vi "PJ1_work.vi"() -> ()   [LabVIEW 2024]
uses:
  C:/Users/Windows 11/Downloads/Control 9.ctl
  <vilib>/Instr/_visa.llb/VISA Configure Serial Port (Instr).vi
  <vilib>/express/express analysis/Spectral/Block/exnSpectralBlock spectral measurements PSD poly.vi
  <vilib>/express/express analysis/Spectral/Block/exnSpectralBlock spectral measurements PSD DDT.vi
  <vilib>/express/express analysis/Spectral/XNode/ExpressSpectralMeasurementsBlockNode.xnode
panel:
  in  "Upper Cut-Off":dbl=40.0
  out "PSD":dynamicdata(graph)
  out "PSD MAX":dbl
  out "Index ที่มากที่สุด":i32
  out "max value":dbl
  out "B 18+1":dbl
  out "N 18+1":dbl
  in  "Aj 18+1":dbl
  out "B 18+1":dbl
  out "PSD 18+1":dbl
  out "B 18":dbl
  out "N 18":dbl
  in  "Aj 18":dbl
  out "B 18":dbl
  out "PSD 18":dbl
  out "B 18-1":dbl
  out "N 18-1":dbl
  in  "Aj 18-1":dbl
  out "B 18-1":dbl
  out "PSD 18-1":dbl
  out "9 Hz":dbl[](array[numeric])
  out "Max Index 9":i32
  out "PSD max 9":dbl
  out "PSD 9-1":dbl
  out "B 9-1":dbl
  in  "Aj 9-1":dbl
  out "N 9-1":dbl
  out "B 9-1":dbl
  out "PSD 9":dbl
  out "B 9":dbl
  in  "Aj 9":dbl
  out "N 9":dbl
  out "B 9":dbl
  out "PSD 9+1":dbl
  out "B 9+1":dbl
  in  "Aj 9+1":dbl
  out "N 9+1":dbl
  out "B 9+1":dbl
  out "8 Hz":dbl[](array[numeric])
  out "Max Index 8":i32
  out "PSD max 8":dbl
  out "B 16+1":dbl
  out "N 16+1":dbl
  in  "Aj  16+1":dbl
  out "B 16+1":dbl
  out "PSD  16+1":dbl
  out "B 16":dbl
  out "N  16":dbl
  in  "Aj  16":dbl
  out "B 16":dbl
  out "PSD  16":dbl
  out "B 16-1":dbl
  out "N  16-1":dbl
  in  "Aj   16-1":dbl
  out "B   16-1":dbl
  out "PSD 16-1":dbl
  out "B 8+1":dbl
  out "N 8+1":dbl
  in  "Aj  8+1":dbl
  out "B  8+1":dbl
  out "PSD 8+1":dbl
  out "B 8":dbl
  out "N  8":dbl
  in  "Aj  8":dbl
  out "B  8":dbl
  out "PSD 8":dbl
  out "B 8-1":dbl
  out "N  8-1":dbl
  in  "Aj  8-1":dbl
  out "B  8-1":dbl
  out "PSD 8-1":dbl
  out "PSD 14+1":dbl
  out "B 14+1":dbl
  in  "Aj 14+1":dbl
  out "N 14+1":dbl
  out "B 14+1":dbl
  out "PSD 14":dbl
  out "B 14":dbl
  in  "Aj 14":dbl
  out "N 14":dbl
  out "B 14":dbl
  out "PSD 14-1":dbl
  out "B 14-1":dbl
  in  "Aj 14-1":dbl
  out "N 14-1":dbl
  out "B 14-1":dbl
  out "PSD7+1":dbl
  out "B7+1":dbl
  in  "Aj7+1":dbl
  out "N7+1":dbl
  out "B7+1":dbl
  out "PSD 7":dbl
  out "B 7":dbl
  in  "Aj 7":dbl
  out "N7":dbl
  out "B7":dbl
  out "7 Hz":dbl[](array[numeric])
  out "Max Index 7":i32
  out "PSD max 7":dbl
  out "PSD 7-1":dbl
  out "B 7-1":dbl
  in  "Aj 7-1":dbl
  out "N7-1":dbl
  out "B7-1":dbl
  out "B12-1":dbl
  out "N12-1":dbl
  in  "Aj 12-1":dbl
  out "B 12-1":dbl
  out "PSD 12-1":dbl
  out "B12":dbl
  out "N12":dbl
  in  "Aj 12":dbl
  out "B12":dbl
  out "PSD 12":dbl
  out "B12+1":dbl
  out "N12+1":dbl
  in  "Aj 12+1":dbl
  out "B 12+1":dbl
  out "PSD 12+1":dbl
  out "B6+1":dbl
  out "N6+1":dbl
  in  "Aj 6+1":dbl
  out "B 6+1":dbl
  out "PSD 6+1":dbl
  out "B6":dbl
  out "N6":dbl
  in  "Aj 6":dbl
  out "B6":dbl
  out "PSD 6":dbl
  out "PSD 6-1":dbl
  out "6 Hz":dbl[](array[numeric])
  out "Max Index 6":i32
  out "PSD max 6":dbl
  out "B 6-1":dbl
  in  "Aj 6-1":dbl
  out "N6-1":dbl
  out "B6-1":dbl
  in  "Baseline":bool
  out "appended array":dbl[][](array[numeric])
  out "Filtered Signal":dynamicdata(graph)
  in  "Lower Cut-Off":dbl=1.0
  out "data":dynamicdata(graph) caption="Raw Data"
  in  "number of samples":i32=1000
  in  "rate":dbl=200.0 min=200.0 max=200.0
  out "?":bool
  out "?":bool
  out "?":bool
  out "?":bool
  out "?":bool
  out "?":bool
  out "?":bool
  out "?":bool
  out "?":bool
  out "?":bool
  out "?":bool=TRUE
  out "?":bool=TRUE
  out "?":bool=TRUE
  out "?":bool=TRUE
  out "?":bool=TRUE
  out "?":bool=TRUE
  out "?":bool=TRUE
  out "?":bool=TRUE
  out "?":bool=TRUE
  out "?":bool=TRUE
  out "?":bool
  out "?":bool
  out "?":bool
  out "?":bool
  out "?":bool
  out "?":bool
  out "?":bool
  out "?":bool
  out "?":bool
  out "?":bool
  out "?":bool=TRUE
  out "?":bool=TRUE
  out "?":bool=TRUE
  out "?":bool=TRUE
  out "?":bool=TRUE
  out "?":bool=TRUE
  out "?":bool=TRUE
  out "?":bool=TRUE
  out "?":bool=TRUE
  out "?":bool=TRUE
  out "?":bool
  out "?":bool
  out "?":bool
  out "?":bool
  out "?":bool
  out "?":bool
  out "?":bool
  out "?":bool
  out "?":bool
  out "?":bool
  out "?":bool=TRUE
  out "?":bool=TRUE
  out "?":bool=TRUE
  out "?":bool=TRUE
  out "?":bool=TRUE
  out "?":bool=TRUE
  out "?":bool=TRUE
  out "?":bool=TRUE
  out "?":bool=TRUE
  out "?":bool=TRUE
  out "?":bool
  out "?":bool
  out "?":bool
  out "?":bool
  out "?":bool
  out "?":bool
  out "?":bool
  out "?":bool
  out "?":bool
  out "?":bool
  out "?":bool=TRUE
  out "?":bool=TRUE
  out "?":bool=TRUE
  out "?":bool=TRUE
  out "?":bool=TRUE
  out "?":bool=TRUE
  out "?":bool=TRUE
  out "?":bool=TRUE
  out "?":bool=TRUE
  out "?":bool=TRUE
  out "9 HZ":bool
  out "8 HZ":bool
  out "6 HZ":bool
  out "7 HZ":bool
  in  "Tab Control":enum32{"TAB 1", "TAB 2", "TAB 3", "TAB 4"}(tab)
  out "555":bool
  in  "MENU 4":bool
  in  "MENU 3":bool
  in  "MENU 2":bool
  in  "MENU":bool
  in  "start":bool
  in  "Text3":bool
  in  "Text2":bool
  in  "Backpage 2":T1
  out "String":string
  in  "Text1":bool
  in  "send":bool
  in  "Back":bool
  in  "1 3":bool
  in  "1 2":bool
  in  "1":bool
  out "String 2":string
  in  "SOS CALLING":bool
  in  "Blank Button 14":bool
  in  "LED":bool
  in  "Blank Button 12":bool
  in  "Back 4":bool
  in  "VISA resource name":refnum<visa-resource-name>
  # "Tel."
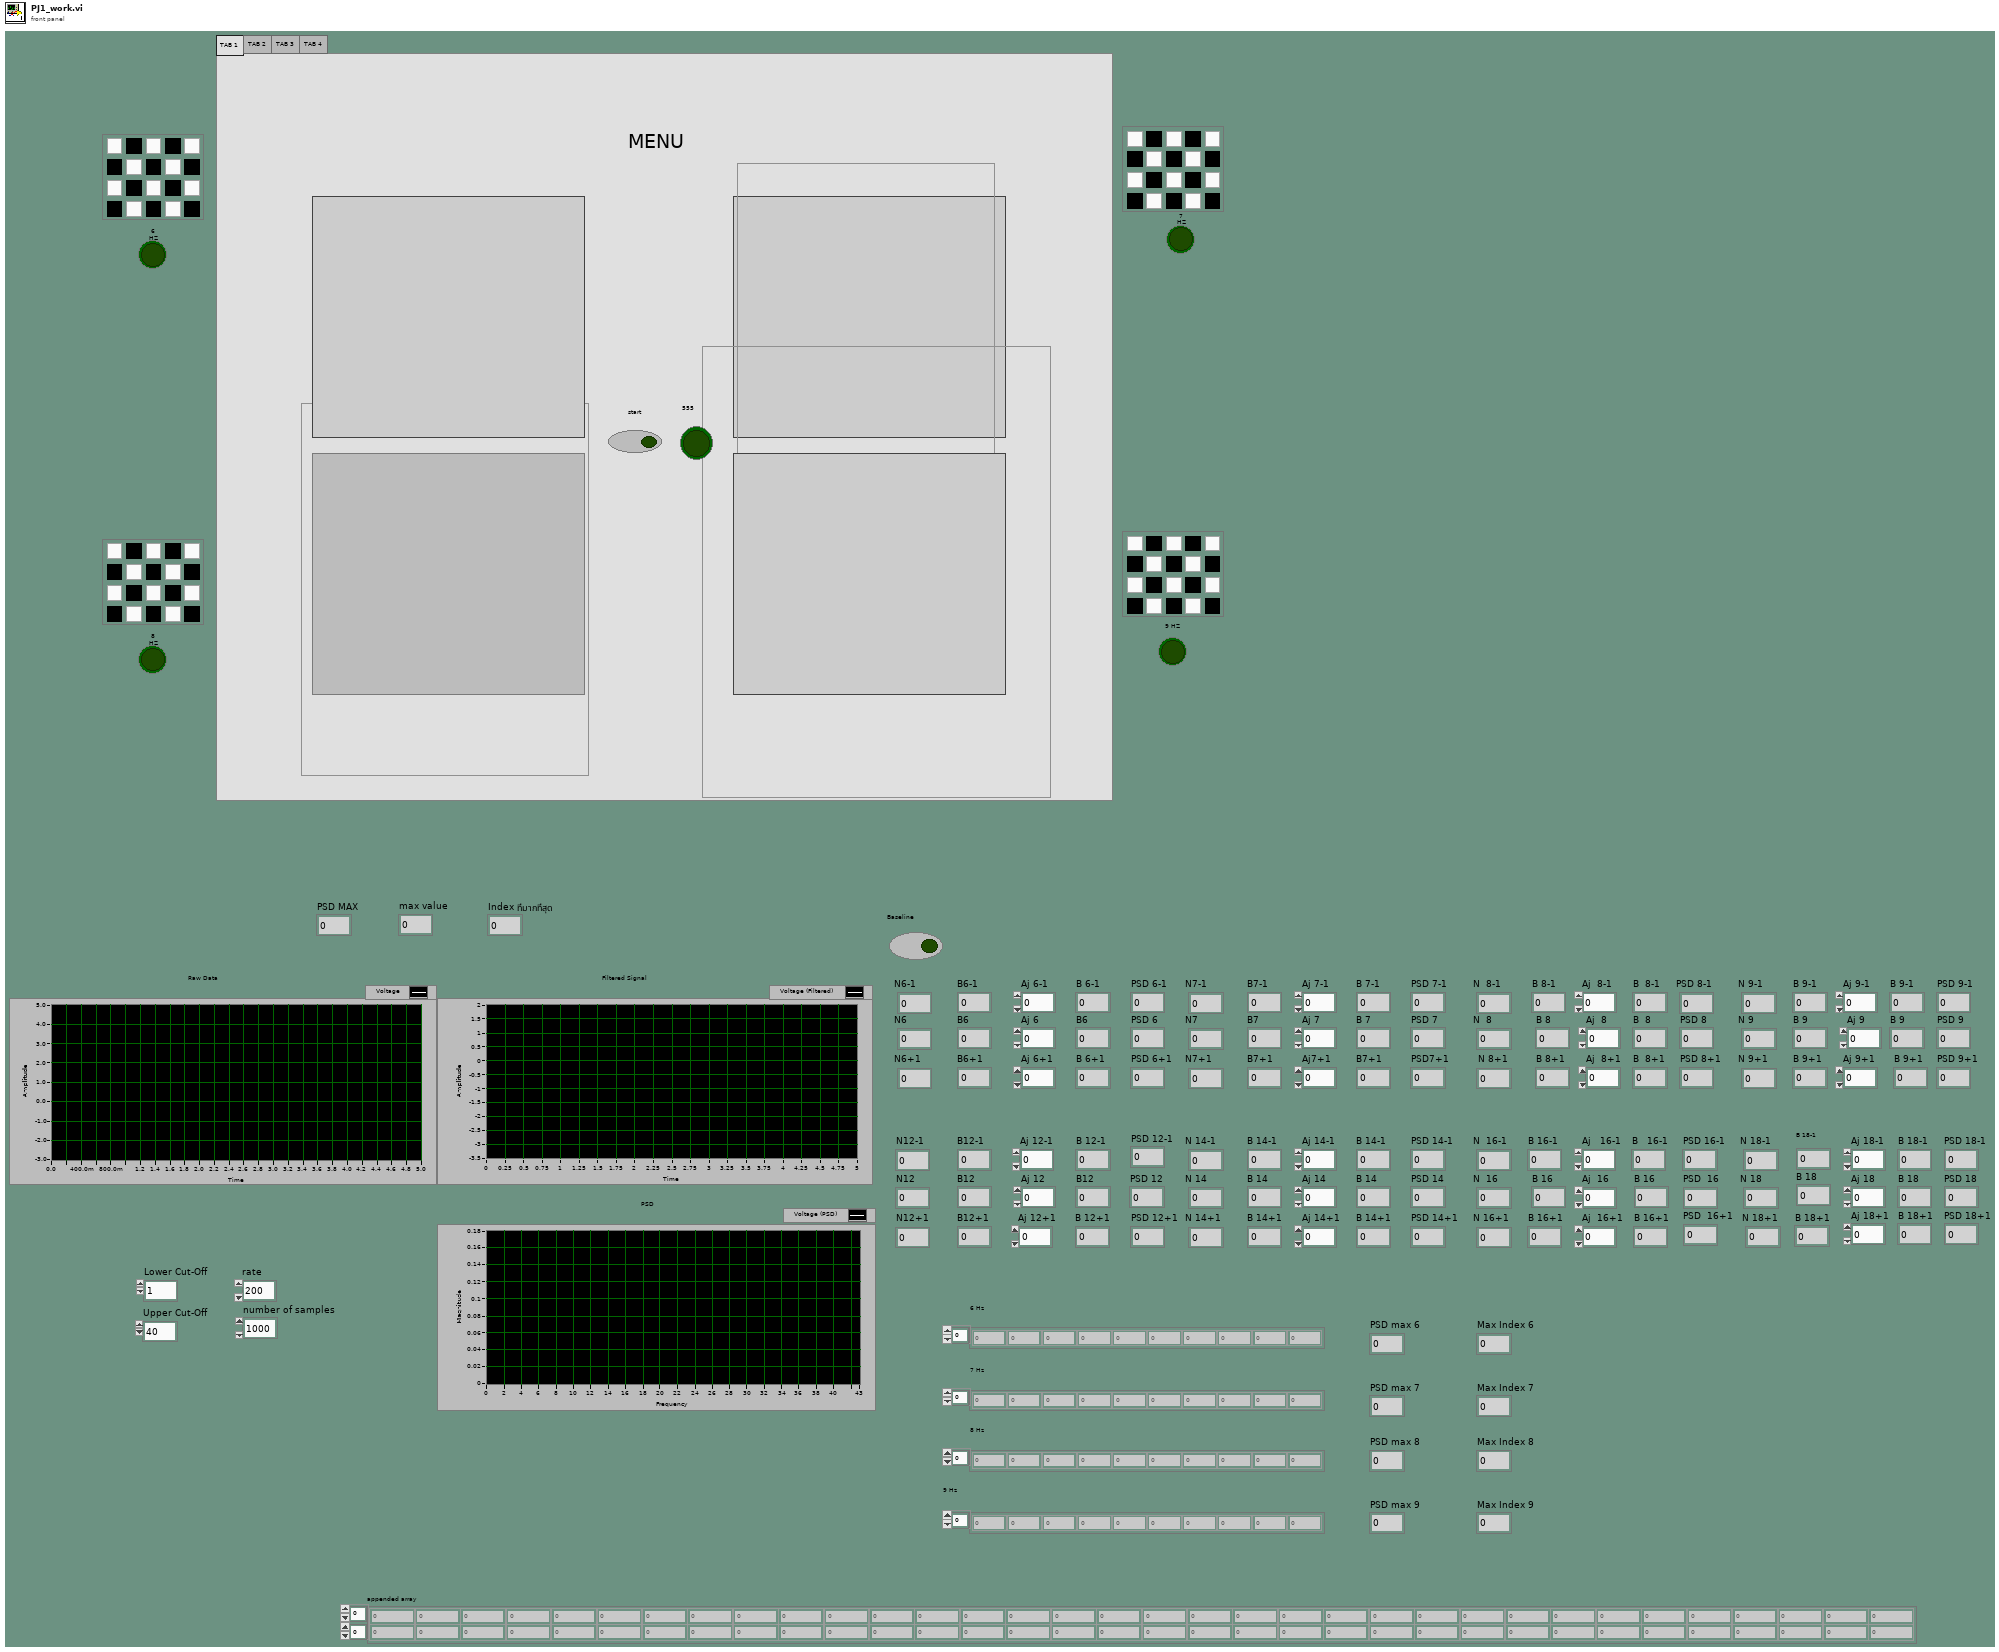
[diagram p1: front panel]
types:
  T1 = typedef "Control 9.ctl" = bool
  T2 = cluster{"averaging mode":u16, "weighting mode":u16, "number of averages":u32}
  T3 = cluster{"dB On (F)":bool, "unwrap phase (F)":bool, "convert to degree (F)":bool}
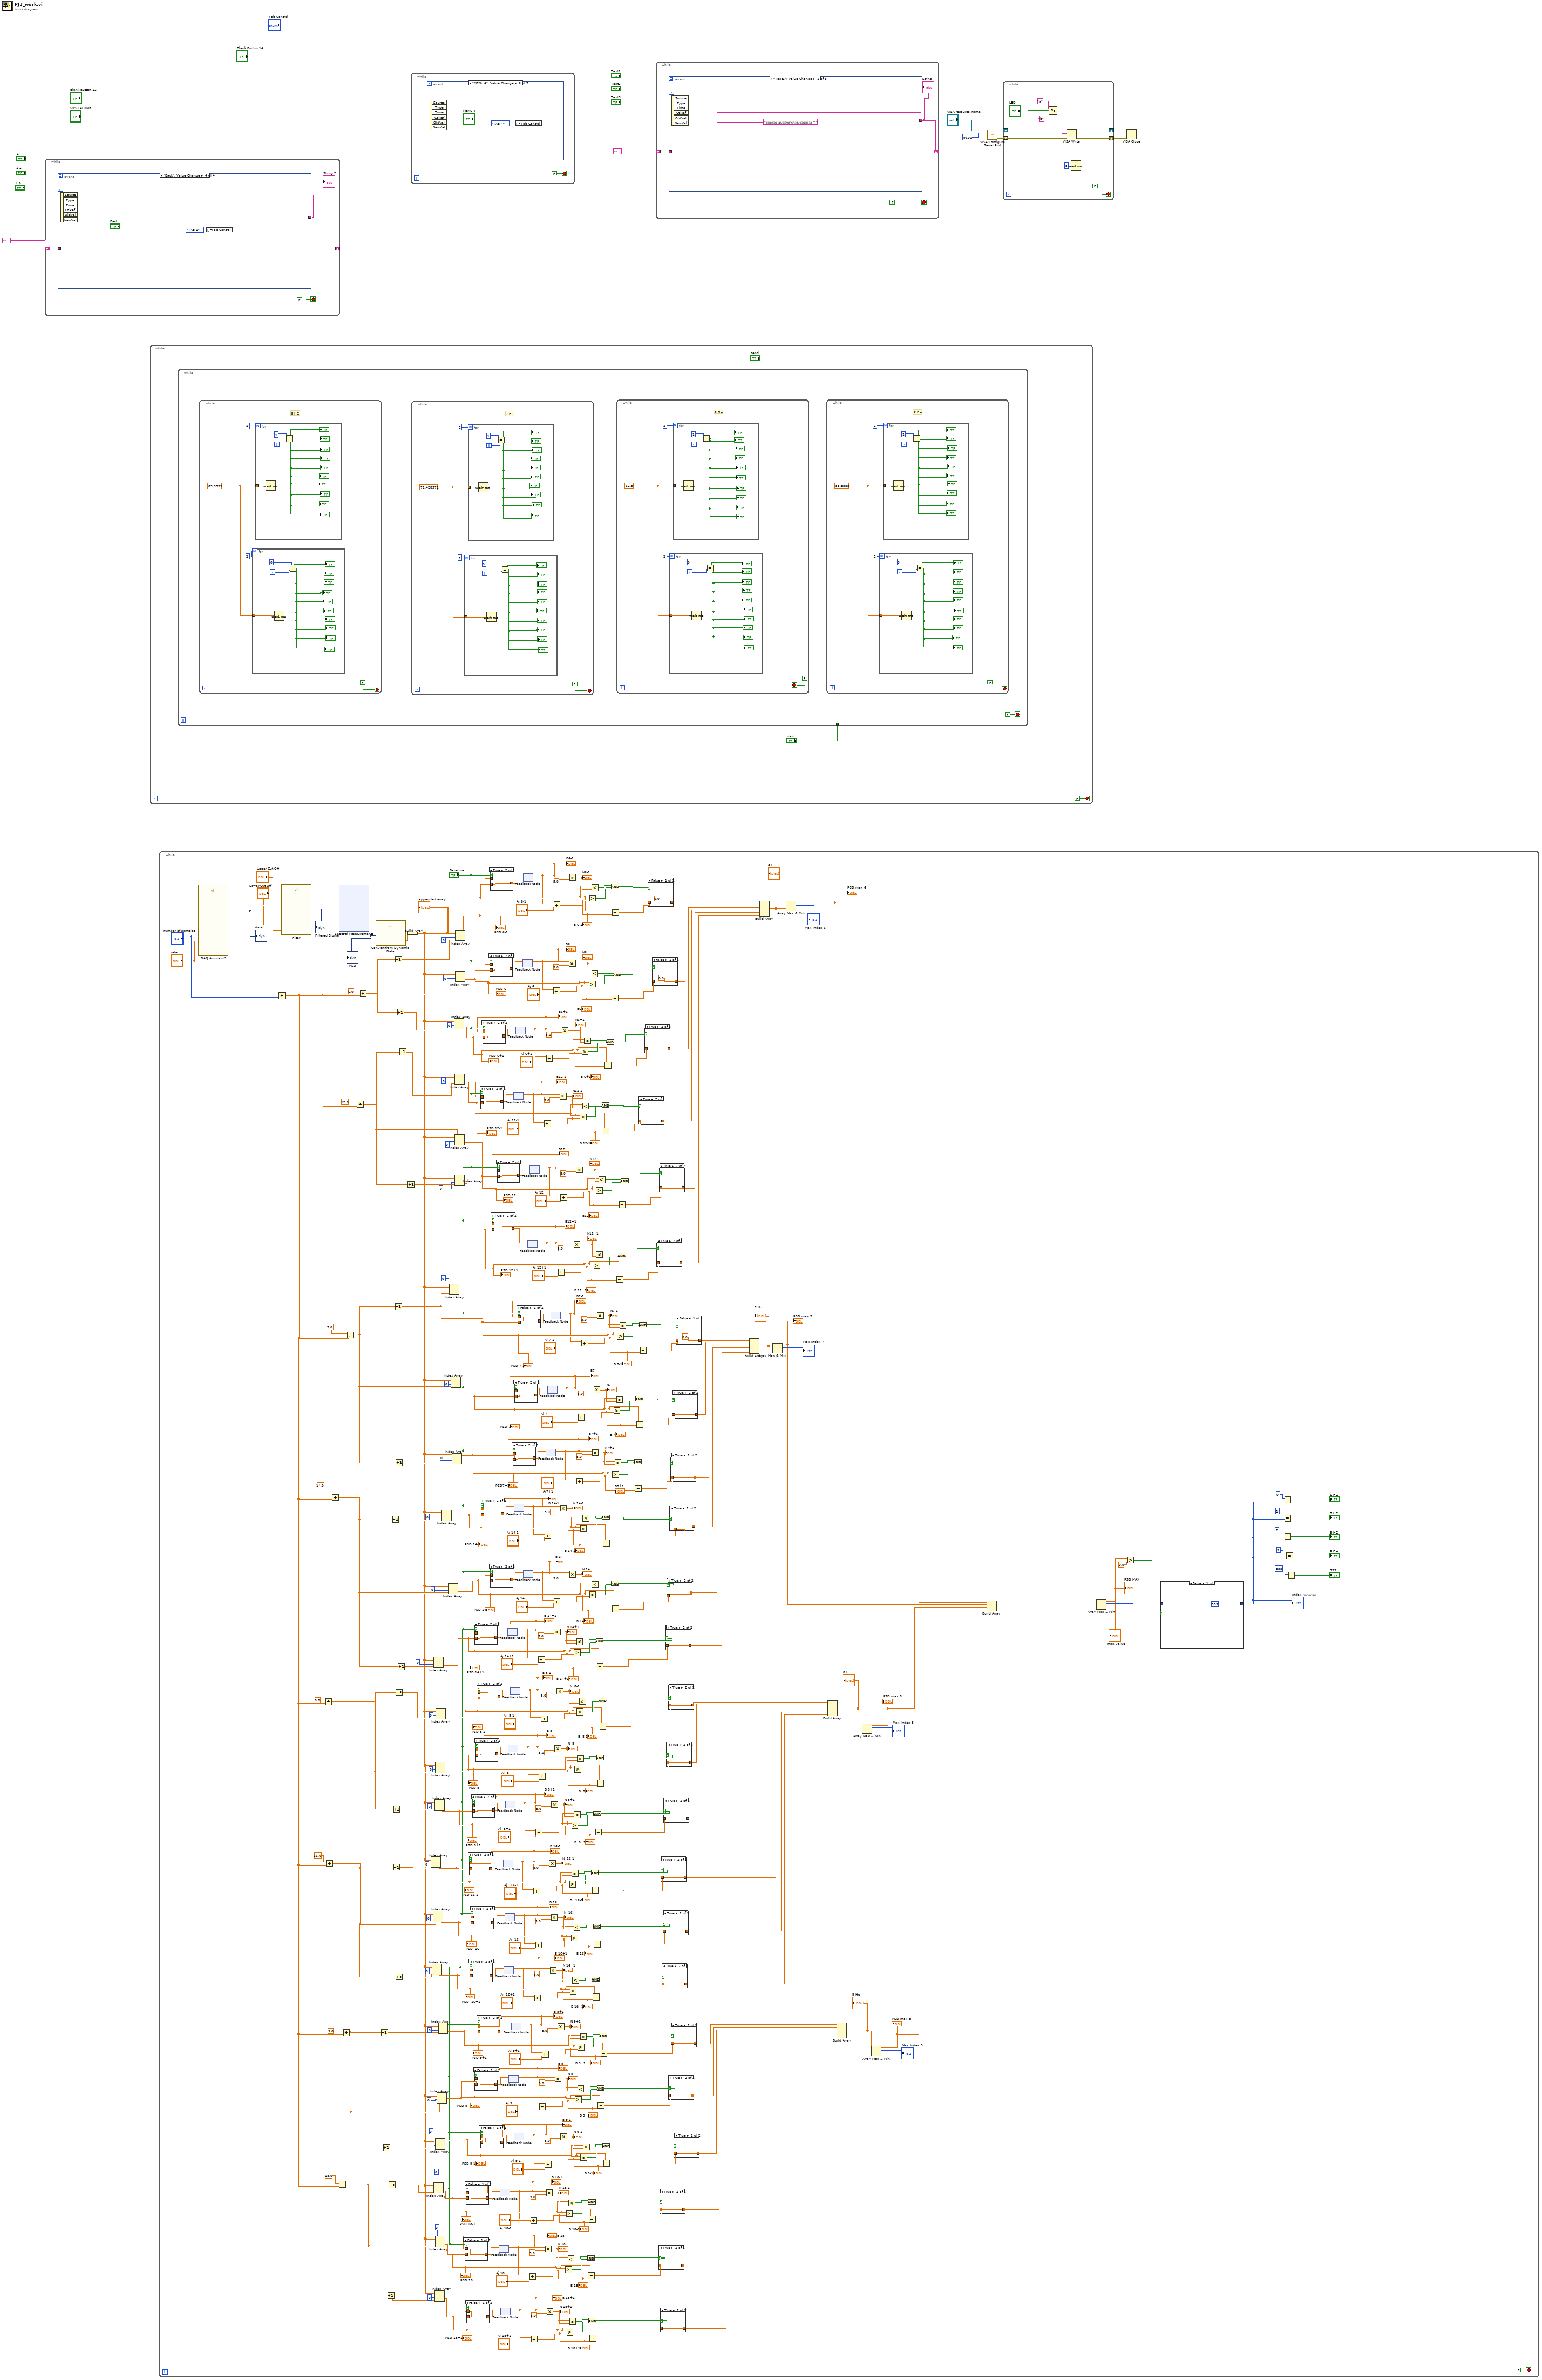
[diagram p0: block diagram]
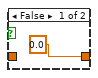
[diagram p3: hidden frame]
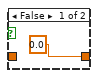
[diagram p5: hidden frame]
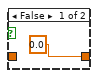
[diagram p7: hidden frame]
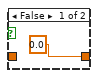
[diagram p9: hidden frame]
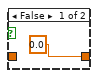
[diagram p11: hidden frame]
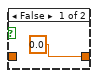
[diagram p13: hidden frame]
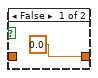
[diagram p15: hidden frame]
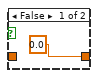
[diagram p17: hidden frame]
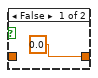
[diagram p19: hidden frame]
diagram:
  n1 = while {
    shift-right: [w9] -> _
    shift-left: "" -> [w11]
    stop <- FALSE stop-if-true
    n2 = event shown="[3] \"Back\": Value Change" {
      selector: _ -> [_ _ _ _]
      dyn-events: _ -> [_ _ _ _]
      timeout: _ -> [_ _ _ _]
      tunnel: w11 -> [_ _ _ _]
      tunnel: ["0622436287" "1669" " 0937529340" _] -> w9
      event "1 2": Value Change {
        n3 = event-data() -> ()  [unwired: 1 in, 6 out]
      }
      event "1": Value Change {
        n4 = event-data() -> ()  [unwired: 1 in, 6 out]
      }
      event "1 3": Value Change {
        n5 = event-data() -> ()  [unwired: 1 in, 6 out]
      }
      event "Back": Value Change {
        n6 = event-data() -> ()  [unwired: 1 in, 6 out]
        n7 = local write "Tab Control"(enum32{"TAB 1", "TAB 2", "TAB 3", "TAB 4"}."TAB 1" ("Tab Control")) -> ()
      }
    }
    "String 2" <- w9
  }
  n8 = while {
    stop <- FALSE stop-if-true
    n9 = while {
      tunnel: "start" -> [_]
      stop <- FALSE stop-if-true
      n10 = while {
        stop <- FALSE stop-if-true
        w56 = 83.3333
        # "6 HZ"
        n11 = for {
          N: 2 -> [_]
          tunnel: w56 -> [w60]
          i -> [w62]
          n12 = Wait (ms)(milliseconds to wait=w60) -> ()  [unwired: 1 out]
          n13 = Equal?(x=0, y=w62) -> (x = y?=→"?" →"?" →"?" →"?" →"?" →"?" →"?" →"?" →"?" →"?":bool)
        }
        n14 = for {
          N: 2 -> [_]
          tunnel: w56 -> [w64]
          i -> [w65]
          n15 = Wait (ms)(milliseconds to wait=w64) -> ()  [unwired: 1 out]
          n16 = Equal?(x=1, y=w65) -> (x = y?=→"?" →"?" →"?" →"?" →"?" →"?" →"?" →"?" →"?" →"?":bool)
        }
      }
      n17 = while {
        stop <- FALSE stop-if-true
        w44 = 71.428571
        # "7 HZ"
        n18 = for {
          N: 2 -> [_]
          tunnel: w44 -> [w48]
          i -> [w50]
          n19 = Wait (ms)(milliseconds to wait=w48) -> ()  [unwired: 1 out]
          n20 = Equal?(x=0, y=w50) -> (x = y?=→"?" →"?" →"?" →"?" →"?" →"?" →"?" →"?" →"?" →"?":bool)
        }
        n21 = for {
          N: 2 -> [_]
          tunnel: w44 -> [w52]
          i -> [w53]
          n22 = Wait (ms)(milliseconds to wait=w52) -> ()  [unwired: 1 out]
          n23 = Equal?(x=1, y=w53) -> (x = y?=→"?" →"?" →"?" →"?" →"?" →"?" →"?" →"?" →"?" →"?":bool)
        }
      }
      n24 = while {
        stop <- FALSE stop-if-true
        w32 = 62.5
        # "8 HZ"
        n25 = for {
          N: 2 -> [_]
          tunnel: w32 -> [w36]
          i -> [w38]
          n26 = Wait (ms)(milliseconds to wait=w36) -> ()  [unwired: 1 out]
          n27 = Equal?(x=0, y=w38) -> (x = y?=→"?" →"?" →"?" →"?" →"?" →"?" →"?" →"?" →"?" →"?":bool)
        }
        n28 = for {
          N: 2 -> [_]
          tunnel: w32 -> [w40]
          i -> [w41]
          n29 = Wait (ms)(milliseconds to wait=w40) -> ()  [unwired: 1 out]
          n30 = Equal?(x=1, y=w41) -> (x = y?=→"?" →"?" →"?" →"?" →"?" →"?" →"?" →"?" →"?" →"?":bool)
        }
      }
      n31 = while {
        stop <- FALSE stop-if-true
        w20 = 55.5555
        # "9 HZ"
        n32 = for {
          N: 2 -> [_]
          tunnel: w20 -> [w24]
          i -> [w26]
          n33 = Wait (ms)(milliseconds to wait=w24) -> ()  [unwired: 1 out]
          n34 = Equal?(x=0, y=w26) -> (x = y?=→"?" →"?" →"?" →"?" →"?" →"?" →"?" →"?" →"?" →"?":bool)
        }
        n35 = for {
          N: 2 -> [_]
          tunnel: w20 -> [w28]
          i -> [w29]
          n36 = Wait (ms)(milliseconds to wait=w28) -> ()  [unwired: 1 out]
          n37 = Equal?(x=1, y=w29) -> (x = y?=→"?" →"?" →"?" →"?" →"?" →"?" →"?" →"?" →"?" →"?":bool)
        }
      }
    }
  }
  n38 = while {
    stop <- FALSE stop-if-true
    n39 = call "DAQ Assistant2"("rate"="rate", "number of samples"="number of samples") -> ("data"=w449:dynamicdata)  [unwired: 15 in, 2 out]
    "data" <- w449
    n40 = Divide(x="rate", y="number of samples") -> (x/y=w156:dbl)
    n41 = call "Filter"("Lower Cut-Off"="Lower Cut-Off", "Upper Cut-Off"="Upper Cut-Off", "Signal"=w449) -> ("Filtered Signal"=w447:dynamicdata)  [unwired: 7 in, 1 out]
    "Filtered Signal" <- w447
    n42 = Divide(x=8.0, y=w156) -> (x/y=w256:dbl)
    n43 = Divide(x=16.0, y=w156) -> (x/y=w208:dbl)
    n44 = Divide(x=14.0, y=w156) -> (x/y=w281:dbl)
    n45 = Divide(x=18.0, y=w156) -> (x/y=w131:dbl)
    n46 = xnode "Spectral Measurements"("Signals"=w447) -> ("PSD"=w93:dynamicdata)  [unwired: 1 in, 1 out]
    "PSD" <- w93
    n47 = Divide(x=9.0, y=w156) -> (x/y=w174:dbl)
    n48 = Divide(x=7.0, y=w156) -> (x/y=w298:dbl)
    n49 = Divide(x=12.0, y=w156) -> (x/y=w367:dbl)
    n50 = Divide(x=6.0, y=w156) -> (x/y=w416:dbl)
    n51 = call "Convert from Dynamic Data"("Dynamic Data Type"=w93) -> ("Array"=w446:dbl[])  [unwired: 3 in]
    n52 = Decrement(x=w174) -> (x-1=w205:dbl)
    n53 = Increment(x=w174) -> (x+1=w173:dbl)
    n54 = Increment(x=w131) -> (x+1=w120:dbl)
    n55 = Decrement(x=w131) -> (x-1=w145:dbl)
    n56 = Decrement(x=w281) -> (x-1=w310:dbl)
    n57 = Increment(x=w256) -> (x+1=w246:dbl)
    n58 = Decrement(x=w208) -> (x-1=w231:dbl)
    n59 = Decrement(x=w416) -> (x-1=w429:dbl)
    n60 = Decrement(x=w298) -> (x-1=w339:dbl)
    "PSD 7-1" <- w339
    n61 = Increment(x=w298) -> (x+1=w324:dbl)
    n62 = Decrement(x=w256) -> (x-1=w269:dbl)
    n63 = Increment(x=w208) -> (x+1=w207:dbl)
    n64 = Increment(x=w416) -> (x+1=w405:dbl)
    n65 = Increment(x=w281) -> (x+1=w287:dbl)
    n66 = Decrement(x=w367) -> (x-1=w372:dbl)
    n67 = Increment(x=w367) -> (x+1=w366:dbl)
    n68 = Build Array(w446) -> (w121:dbl[][])
    "appended array" <- w121
    n69 = Index Array(array=w121, index (row)=0, index (col)=w231) -> (element=w242:dbl)
    "PSD 16-1" <- w242
    n70 = Index Array(array=w121, index (row)=0 ("disabled index (row)"), index (col)=w207) -> (element=w219:dbl)
    "PSD  16+1" <- w219
    n71 = Index Array(array=w121, index (row)=0 ("disabled index (row)"), index (col)=w208) -> (element=w221:dbl)
    "PSD  16" <- w221
    n72 = Index Array(array=w121, index (row)=0, index (col)=w287) -> (element=w288:dbl)
    "PSD 14+1" <- w288
    n73 = Index Array(array=w121, index (row)=0 ("disabled index (row)"), index (col)=w145) -> (element=w143:dbl)
    "PSD 18-1" <- w143
    n74 = Index Array(array=w121, index (row)=0, index (col)=w246) -> (element=w244:dbl)
    "PSD 8+1" <- w244
    n75 = Index Array(array=w121, index (row)=0 ("disabled index (row)"), index (col)=w120) -> (element=w117:dbl)
    "PSD 18+1" <- w117
    n76 = Index Array(array=w121, index (row)=0, index (col)=w173) -> (element=w162:dbl)
    "PSD 9-1" <- w162
    n77 = Index Array(array=w121, index (row)=0, index (col)=w256) -> (element=w267:dbl)
    "PSD 8" <- w267
    n78 = Index Array(array=w121, index (row)=0 ("disabled index (row)"), index (col)=w131) -> (element=w132:dbl)
    "PSD 18" <- w132
    n79 = Index Array(array=w121, index (row)=0, index (col)=w269) -> (element=w268:dbl)
    "PSD 8-1" <- w268
    n80 = Index Array(array=w121, index (row)=0, index (col)=w174) -> (element=w175:dbl)
    "PSD 9" <- w175
    n81 = Index Array(array=w121, index (row)=0, index (col)=w205) -> (element=w186:dbl)
    "PSD 9+1" <- w186
    n82 = Index Array(array=w121, index (row)=0, index (col)=w310) -> (element=w312:dbl)
    "PSD 14-1" <- w312
    n83 = Index Array(array=w121, index (row)=0, index (col)=w281) -> (element=w299:dbl)
    "PSD 14" <- w299
    n84 = Index Array(array=w121, index (row)=0, index (col)=w339) -> ()  [unwired: 1 out]
    n85 = Index Array(array=w121, index (row)=0 ("disabled index (row)"), index (col)=w298) -> (element=w336:dbl)
    "PSD 7" <- w336
    n86 = Index Array(array=w121, index (row)=0, index (col)=w324) -> (element=w325:dbl)
    "PSD7+1" <- w325
    n87 = Index Array(array=w121, index (row)=0 ("disabled index (row)"), index (col)=w405) -> (element=w403:dbl)
    "PSD 6+1" <- w403
    n88 = Index Array(array=w121, index (row)=0, index (col)=w372) -> (element=w371:dbl)
    "PSD 12-1" <- w371
    n89 = Index Array(array=w121, index (row)=0 ("disabled index (row)"), index (col)=w367) -> (element=w368:dbl)
    "PSD 12" <- w368
    n90 = Index Array(array=w121, index (row)=0 ("disabled index (row)"), index (col)=w366) -> (element=w364:dbl)
    "PSD 12+1" <- w364
    n91 = Index Array(array=w121, index (row)=0, index (col)=w416) -> (element=w417:dbl)
    "PSD 6" <- w417
    n92 = Index Array(array=w121, index (row)=0, index (col)=w429) -> (element=w436:dbl)
    "PSD 6-1" <- w436
    n93 = feedback #1() -> (w69:dbl)  [unwired: 1 in]
    "B 18" <- w69
    n94 = case shown="False" "Baseline" {
      tunnel: w132 -> [_ w459]
      tunnel: [w458 w459] -> w134
      tunnel: w69 -> [w458 _]
      frame False {
      }
      frame True {
      }
    }
    n95 = feedback-in #1(w134) -> ()
    n96 = feedback #2() -> (w70:dbl)  [unwired: 1 in]
    "B 18-1" <- w70
    n97 = case shown="False" "Baseline" {
      tunnel: w143 -> [_ w463]
      tunnel: [w462 w463] -> w154
      tunnel: w70 -> [w462 _]
      frame False {
      }
      frame True {
      }
    }
    n98 = feedback-in #2(w154) -> ()
    n99 = feedback #3() -> (w68:dbl)  [unwired: 1 in]
    "B 18+1" <- w68
    n100 = case shown="False" "Baseline" {
      tunnel: w117 -> [_ w455]
      tunnel: [w454 w455] -> w130
      tunnel: w68 -> [w454 _]
      frame False {
      }
      frame True {
      }
    }
    n101 = feedback-in #3(w130) -> ()
    n102 = feedback #4() -> (w76:dbl)  [unwired: 1 in]
    "B 16-1" <- w76
    n103 = case shown="True" "Baseline" {
      tunnel: w242 -> [_ w487]
      tunnel: [w486 w487] -> w232
      tunnel: w76 -> [w486 _]
      frame False {
      }
      frame True {
      }
    }
    n104 = feedback-in #4(w232) -> ()
    n105 = feedback #5() -> (w74:dbl)  [unwired: 1 in]
    "B 16+1" <- w74
    n106 = case shown="True" "Baseline" {
      tunnel: w219 -> [_ w479]
      tunnel: [w478 w479] -> w210
      tunnel: w74 -> [w478 _]
      frame False {
      }
      frame True {
      }
    }
    n107 = feedback-in #5(w210) -> ()
    n108 = feedback #6() -> (w75:dbl)  [unwired: 1 in]
    "B 16" <- w75
    n109 = case shown="True" "Baseline" {
      tunnel: w221 -> [_ w483]
      tunnel: [w482 w483] -> w230
      tunnel: w75 -> [w482 _]
      frame False {
      }
      frame True {
      }
    }
    n110 = feedback-in #6(w230) -> ()
    n111 = feedback #7() -> (w77:dbl)  [unwired: 1 in]
    "B 8+1" <- w77
    n112 = case shown="True" "Baseline" {
      tunnel: w244 -> [_ w491]
      tunnel: [w490 w491] -> w255
      tunnel: w77 -> [w490 _]
      frame False {
      }
      frame True {
      }
    }
    n113 = feedback-in #7(w255) -> ()
    n114 = feedback #8() -> (w80:dbl)  [unwired: 1 in]
    "B 14+1" <- w80
    n115 = case shown="True" "Baseline" {
      tunnel: w288 -> [_ w503]
      tunnel: [w502 w503] -> w289
      tunnel: w80 -> [w502 _]
      frame False {
      }
      frame True {
      }
    }
    n116 = feedback-in #8(w289) -> ()
    n117 = feedback #9() -> (w78:dbl)  [unwired: 1 in]
    "B 8" <- w78
    n118 = case shown="True" "Baseline" {
      tunnel: w267 -> [_ w495]
      tunnel: [w494 w495] -> w258
      tunnel: w78 -> [w494 _]
      frame False {
      }
      frame True {
      }
    }
    n119 = feedback-in #9(w258) -> ()
    n120 = feedback #10() -> (w72:dbl)  [unwired: 1 in]
    "B 9" <- w72
    n121 = case shown="False" "Baseline" {
      tunnel: w175 -> [_ w471]
      tunnel: [w470 w471] -> w176
      tunnel: w72 -> [w470 _]
      frame False {
      }
      frame True {
      }
    }
    n122 = feedback-in #10(w176) -> ()
    n123 = feedback #11() -> (w79:dbl)  [unwired: 1 in]
    "B 8-1" <- w79
    n124 = case shown="True" "Baseline" {
      tunnel: w268 -> [_ w499]
      tunnel: [w498 w499] -> w279
      tunnel: w79 -> [w498 _]
      frame False {
      }
      frame True {
      }
    }
    n125 = feedback-in #11(w279) -> ()
    n126 = feedback #12() -> (w73:dbl)  [unwired: 1 in]
    "B 9+1" <- w73
    n127 = case shown="True" "Baseline" {
      tunnel: w186 -> [_ w475]
      tunnel: [w474 w475] -> w187
      tunnel: w73 -> [w474 _]
      frame False {
      }
      frame True {
      }
    }
    n128 = feedback-in #12(w187) -> ()
    n129 = feedback #13() -> (w88:dbl)  [unwired: 1 in]
    "B12-1" <- w88
    n130 = case shown="True" "Baseline" {
      tunnel: w371 -> [_ w535]
      tunnel: [w534 w535] -> w383
      tunnel: w88 -> [w534 _]
      frame False {
      }
      frame True {
      }
    }
    n131 = feedback-in #13(w383) -> ()
    n132 = feedback #14() -> (w82:dbl)  [unwired: 1 in]
    "B 14-1" <- w82
    n133 = case shown="True" "Baseline" {
      tunnel: w312 -> [_ w511]
      tunnel: [w510 w511] -> w313
      tunnel: w82 -> [w510 _]
      frame False {
      }
      frame True {
      }
    }
    n134 = feedback-in #14(w313) -> ()
    n135 = feedback #15() -> (w71:dbl)  [unwired: 1 in]
    "B 9-1" <- w71
    n136 = case shown="False" "Baseline" {
      tunnel: w162 -> [_ w467]
      tunnel: [w466 w467] -> w163
      tunnel: w71 -> [w466 _]
      frame False {
      }
      frame True {
      }
    }
    n137 = feedback-in #15(w163) -> ()
    n138 = feedback #16() -> (w89:dbl)  [unwired: 1 in]
    "B6+1" <- w89
    n139 = case shown="True" "Baseline" {
      tunnel: w403 -> [_ w539]
      tunnel: [w538 w539] -> w406
      tunnel: w89 -> [w538 _]
      frame False {
      }
      frame True {
      }
    }
    n140 = feedback-in #16(w406) -> ()
    n141 = feedback #17() -> (w90:dbl)  [unwired: 1 in]
    "B6" <- w90
    n142 = case shown="True" "Baseline" {
      tunnel: w417 -> [_ w543]
      tunnel: [w542 w543] -> w427
      tunnel: w90 -> [w542 _]
      frame False {
      }
      frame True {
      }
    }
    n143 = feedback-in #17(w427) -> ()
    n144 = feedback #18() -> (w91:dbl)  [unwired: 1 in]
    "B6-1" <- w91
    n145 = case shown="True" "Baseline" {
      tunnel: w436 -> [_ w547]
      tunnel: [w546 w547] -> w428
      tunnel: w91 -> [w546 _]
      frame False {
      }
      frame True {
      }
    }
    n146 = feedback-in #18(w428) -> ()
    n147 = feedback #19() -> (w81:dbl)  [unwired: 1 in]
    "B 14" <- w81
    n148 = case shown="True" "Baseline" {
      tunnel: w299 -> [_ w507]
      tunnel: [w506 w507] -> w301
      tunnel: w81 -> [w506 _]
      frame False {
      }
      frame True {
      }
    }
    n149 = feedback-in #19(w301) -> ()
    n150 = feedback #20() -> (w86:dbl)  [unwired: 1 in]
    "B12+1" <- w86
    n151 = case shown="True" "Baseline" {
      tunnel: w364 -> [_ w527]
      tunnel: [w526 w527] -> w401
      tunnel: w86 -> [w526 _]
      frame False {
      }
      frame True {
      }
    }
    n152 = feedback-in #20(w401) -> ()
    n153 = Add(x=w69, y="Aj 18") -> (x+y=w138:dbl)
    "B 18" <- w138
    n154 = Add(x=w70, y="Aj 18-1") -> (x+y=w150:dbl)
    "B 18-1" <- w150
    n155 = Add(x=w68, y="Aj 18+1") -> (x+y=w126:dbl)
    "B 18+1" <- w126
    n156 = feedback #21() -> (w87:dbl)  [unwired: 1 in]
    "B12" <- w87
    n157 = case shown="True" "Baseline" {
      tunnel: w368 -> [_ w531]
      tunnel: [w530 w531] -> w384
      tunnel: w87 -> [w530 _]
      frame False {
      }
      frame True {
      }
    }
    n158 = feedback-in #21(w384) -> ()
    n159 = Add(x=w76, y="Aj   16-1") -> (x+y=w236:dbl)
    "B   16-1" <- w236
    n160 = Add(x=w74, y="Aj  16+1") -> (x+y=w214:dbl)
    "B 16+1" <- w214
    n161 = Add(x=w75, y="Aj  16") -> (x+y=w226:dbl)
    "B 16" <- w226
    n162 = Add(x=w77, y="Aj  8+1") -> (x+y=w251:dbl)
    "B  8+1" <- w251
    n163 = Add(x=w80, y="Aj 14+1") -> (x+y=w293:dbl)
    "B 14+1" <- w293
    n164 = Add(x=w78, y="Aj  8") -> (x+y=w262:dbl)
    "B  8" <- w262
    n165 = Add(x=w72, y="Aj 9") -> (x+y=w180:dbl)
    "B 9" <- w180
    n166 = Add(x=w79, y="Aj  8-1") -> (x+y=w275:dbl)
    "B  8-1" <- w275
    n167 = Add(x=w73, y="Aj 9+1") -> (x+y=w191:dbl)
    "B 9+1" <- w191
    n168 = Add(x=w88, y="Aj 12-1") -> (x+y=w379:dbl)
    "B 12-1" <- w379
    n169 = Add(x=w82, y="Aj 14-1") -> (x+y=w317:dbl)
    "B 14-1" <- w317
    n170 = Add(x=w71, y="Aj 9-1") -> (x+y=w167:dbl)
    "B 9-1" <- w167
    n171 = Multiply(x=w69, y=5.0) -> (x*y=w141:dbl)
    "N 18" <- w141
    n172 = Add(x=w89, y="Aj 6+1") -> (x+y=w410:dbl)
    "B 6+1" <- w410
    n173 = Multiply(x=w70, y=5.0) -> (x*y=w147:dbl)
    "N 18-1" <- w147
    n174 = Multiply(x=w68, y=5.0) -> (x*y=w123:dbl)
    "N 18+1" <- w123
    n175 = feedback #22() -> (w83:dbl)  [unwired: 1 in]
    "B7+1" <- w83
    n176 = case shown="True" "Baseline" {
      tunnel: w325 -> [_ w515]
      tunnel: [w514 w515] -> w327
      tunnel: w83 -> [w514 _]
      frame False {
      }
      frame True {
      }
    }
    n177 = feedback-in #22(w327) -> ()
    n178 = feedback #23() -> (w84:dbl)  [unwired: 1 in]
    "B7" <- w84
    n179 = case shown="True" "Baseline" {
      tunnel: w336 -> [_ w519]
      tunnel: [w518 w519] -> w340
      tunnel: w84 -> [w518 _]
      frame False {
      }
      frame True {
      }
    }
    n180 = feedback-in #23(w340) -> ()
    n181 = Multiply(x=w76, y=5.0) -> (x*y=w239:dbl)
    "N  16-1" <- w239
    n182 = Multiply(x=w74, y=5.0) -> (x*y=w217:dbl)
    "N 16+1" <- w217
    n183 = Multiply(x=w75, y=5.0) -> (x*y=w223:dbl)
    "N  16" <- w223
    n184 = Multiply(x=w77, y=5.0) -> (x*y=w248:dbl)
    "N 8+1" <- w248
    n185 = feedback #24() -> (w85:dbl)  [unwired: 1 in]
    "B7-1" <- w85
    n186 = case shown="False" "Baseline" {
      tunnel: w339 -> [_ w523]
      tunnel: [w522 w523] -> w353
      tunnel: w85 -> [w522 _]
      frame False {
      }
      frame True {
      }
    }
    n187 = feedback-in #24(w353) -> ()
    n188 = Add(x=w90, y="Aj 6") -> (x+y=w423:dbl)
    "B6" <- w423
    n189 = Add(x=w91, y="Aj 6-1") -> (x+y=w437:dbl)
    "B 6-1" <- w437
    n190 = Add(x=w81, y="Aj 14") -> (x+y=w305:dbl)
    "B 14" <- w305
    n191 = Multiply(x=w80, y=5.0) -> (x*y=w296:dbl)
    "N 14+1" <- w296
    n192 = Multiply(x=w78, y=5.0) -> (x*y=w265:dbl)
    "N  8" <- w265
    n193 = Multiply(x=w72, y=5.0) -> (x*y=w183:dbl)
    "N 9" <- w183
    n194 = Multiply(x=w79, y=5.0) -> (x*y=w272:dbl)
    "N  8-1" <- w272
    n195 = Multiply(x=w73, y=5.0) -> (x*y=w194:dbl)
    "N 9+1" <- w194
    n196 = Add(x=w86, y="Aj 12+1") -> (x+y=w397:dbl)
    "B 12+1" <- w397
    n197 = Multiply(x=w88, y=5.0) -> (x*y=w376:dbl)
    "N12-1" <- w376
    n198 = Multiply(x=w82, y=5.0) -> (x*y=w320:dbl)
    "N 14-1" <- w320
    n199 = Add(x=w87, y="Aj 12") -> (x+y=w388:dbl)
    "B12" <- w388
    n200 = Multiply(x=w71, y=5.0) -> (x*y=w170:dbl)
    "N 9-1" <- w170
    n201 = Multiply(x=w89, y=5.0) -> (x*y=w413:dbl)
    "N6+1" <- w413
    n202 = Greater?(x=w132, y=w138) -> (0:w139:bool)
    n203 = Greater?(x=w143, y=w150) -> (0:w149:bool)
    n204 = Greater?(x=w117, y=w126) -> (0:w125:bool)
    n205 = Less?(x=w132, y=w141) -> (x < y?=w140:bool)
    n206 = Less?(x=w143, y=w147) -> (x < y?=w148:bool)
    n207 = Multiply(x=w90, y=5.0) -> (x*y=w420:dbl)
    "N6" <- w420
    n208 = Multiply(x=w91, y=5.0) -> (x*y=w440:dbl)
    "N6-1" <- w440
    n209 = Multiply(x=w81, y=5.0) -> (x*y=w308:dbl)
    "N 14" <- w308
    n210 = Greater?(x=w242, y=w236) -> (0:w237:bool)
    n211 = Less?(x=w117, y=w123) -> (x < y?=w124:bool)
    n212 = Greater?(x=w219, y=w214) -> (0:w215:bool)
    n213 = Greater?(x=w221, y=w226) -> (0:w225:bool)
    n214 = Greater?(x=w244, y=w251) -> (0:w250:bool)
    n215 = Less?(x=w242, y=w239) -> (x < y?=w238:bool)
    n216 = Less?(x=w219, y=w217) -> (x < y?=w216:bool)
    n217 = Multiply(x=w86, y=5.0) -> (x*y=w394:dbl)
    "N12+1" <- w394
    n218 = Less?(x=w221, y=w223) -> (x < y?=w224:bool)
    n219 = Greater?(x=w288, y=w293) -> (0:w294:bool)
    n220 = Less?(x=w244, y=w248) -> (x < y?=w249:bool)
    n221 = Greater?(x=w267, y=w262) -> (0:w263:bool)
    n222 = Greater?(x=w175, y=w180) -> (0:w181:bool)
    n223 = Multiply(x=w87, y=5.0) -> (x*y=w391:dbl)
    "N12" <- w391
    n224 = Add(x=w83, y="Aj7+1") -> (x+y=w331:dbl)
    "B7+1" <- w331
    n225 = Less?(x=w288, y=w296) -> (x < y?=w295:bool)
    n226 = Greater?(x=w268, y=w275) -> (0:w274:bool)
    n227 = Less?(x=w267, y=w265) -> (x < y?=w264:bool)
    n228 = Less?(x=w175, y=w183) -> (x < y?=w182:bool)
    n229 = Greater?(x=w186, y=w191) -> (0:w192:bool)
    n230 = Add(x=w84, y="Aj 7") -> (x+y=w344:dbl)
    "B 7" <- w344
    n231 = Less?(x=w268, y=w272) -> (x < y?=w273:bool)
    n232 = Greater?(x=w371, y=w379) -> (0:w378:bool)
    n233 = Greater?(x=w312, y=w317) -> (0:w318:bool)
    n234 = Less?(x=w186, y=w194) -> (x < y?=w193:bool)
    n235 = Greater?(x=w162, y=w167) -> (0:w168:bool)
    n236 = Add(x=w85, y="Aj 7-1") -> (x+y=w357:dbl)
    "B 7-1" <- w357
    n237 = Greater?(x=w403, y=w410) -> (0:w411:bool)
    n238 = Less?(x=w371, y=w376) -> (x < y?=w377:bool)
    n239 = Less?(x=w312, y=w320) -> (x < y?=w319:bool)
    n240 = Less?(x=w162, y=w170) -> (x < y?=w169:bool)
    n241 = Less?(x=w403, y=w413) -> (x < y?=w412:bool)
    n242 = And(x=w140, y=w139) -> (x .and. y?=w137:bool)
    n243 = Subtract(x=w132, y=w138) -> (x-y=w136:dbl)
    n244 = And(x=w148, y=w149) -> (x .and. y?=w151:bool)
    n245 = Greater?(x=w417, y=w423) -> (0:w422:bool)
    n246 = Subtract(x=w143, y=w150) -> (x-y=w152:dbl)
    n247 = Greater?(x=w436, y=w437) -> (0:w438:bool)
    n248 = Greater?(x=w299, y=w305) -> (0:w306:bool)
    n249 = And(x=w124, y=w125) -> (x .and. y?=w127:bool)
    n250 = Subtract(x=w117, y=w126) -> (x-y=w128:dbl)
    n251 = Less?(x=w417, y=w420) -> (x < y?=w421:bool)
    n252 = Less?(x=w436, y=w440) -> (x < y?=w439:bool)
    n253 = Less?(x=w299, y=w308) -> (x < y?=w307:bool)
    n254 = And(x=w238, y=w237) -> (x .and. y?=w235:bool)
    n255 = Multiply(x=w83, y=5.0) -> (x*y=w334:dbl)
    "N7+1" <- w334
    n256 = Subtract(x=w242, y=w236) -> (x-y=w234:dbl)
    n257 = And(x=w216, y=w215) -> (x .and. y?=w213:bool)
    n258 = Subtract(x=w219, y=w214) -> (x-y=w212:dbl)
    n259 = Greater?(x=w364, y=w397) -> (0:w396:bool)
    n260 = Multiply(x=w84, y=5.0) -> (x*y=w347:dbl)
    "N7" <- w347
    n261 = And(x=w224, y=w225) -> (x .and. y?=w227:bool)
    n262 = And(x=w249, y=w250) -> (x .and. y?=w252:bool)
    n263 = Subtract(x=w221, y=w226) -> (x-y=w228:dbl)
    n264 = Subtract(x=w244, y=w251) -> (x-y=w253:dbl)
    n265 = Greater?(x=w368, y=w388) -> (0:w389:bool)
    n266 = Less?(x=w364, y=w394) -> (x < y?=w395:bool)
    n267 = And(x=w295, y=w294) -> (x .and. y?=w292:bool)
    n268 = Subtract(x=w288, y=w293) -> (x-y=w291:dbl)
    n269 = Multiply(x=w85, y=5.0) -> (x*y=w360:dbl)
    "N7-1" <- w360
    n270 = And(x=w264, y=w263) -> (x .and. y?=w261:bool)
    n271 = Subtract(x=w267, y=w262) -> (x-y=w260:dbl)
    n272 = And(x=w182, y=w181) -> (x .and. y?=w179:bool)
    n273 = Subtract(x=w175, y=w180) -> (x-y=w178:dbl)
    n274 = Less?(x=w368, y=w391) -> (x < y?=w390:bool)
    n275 = And(x=w273, y=w274) -> (x .and. y?=w276:bool)
    n276 = Subtract(x=w268, y=w275) -> (x-y=w277:dbl)
    n277 = And(x=w193, y=w192) -> (x .and. y?=w190:bool)
    n278 = Subtract(x=w186, y=w191) -> (x-y=w189:dbl)
    n279 = And(x=w377, y=w378) -> (x .and. y?=w380:bool)
    n280 = Subtract(x=w371, y=w379) -> (x-y=w381:dbl)
    n281 = And(x=w319, y=w318) -> (x .and. y?=w316:bool)
    n282 = Subtract(x=w312, y=w317) -> (x-y=w315:dbl)
    n283 = And(x=w169, y=w168) -> (x .and. y?=w166:bool)
    n284 = Subtract(x=w162, y=w167) -> (x-y=w165:dbl)
    n285 = Subtract(x=w403, y=w410) -> (x-y=w408:dbl)
    n286 = And(x=w412, y=w411) -> (x .and. y?=w409:bool)
    n287 = And(x=w439, y=w438) -> (x .and. y?=w435:bool)
    n288 = Subtract(x=w417, y=w423) -> (x-y=w425:dbl)
    n289 = And(x=w307, y=w306) -> (x .and. y?=w304:bool)
    n290 = Subtract(x=w436, y=w437) -> (x-y=w434:dbl)
    n291 = Greater?(x=w325, y=w331) -> (0:w332:bool)
    n292 = Subtract(x=w299, y=w305) -> (x-y=w303:dbl)
    n293 = Greater?(x=w336, y=w344) -> (0:w345:bool)
    n294 = And(x=w421, y=w422) -> (x .and. y?=w424:bool)
    n295 = Less?(x=w325, y=w334) -> (x < y?=w333:bool)
    n296 = Less?(x=w336, y=w347) -> (x < y?=w346:bool)
    n297 = Subtract(x=w364, y=w397) -> (x-y=w399:dbl)
    n298 = Greater?(x=w339, y=w357) -> (0:w358:bool)
    n299 = Subtract(x=w368, y=w388) -> (x-y=w386:dbl)
    n300 = And(x=w395, y=w396) -> (x .and. y?=w398:bool)
    n301 = Less?(x=w339, y=w360) -> (x < y?=w359:bool)
    n302 = And(x=w390, y=w389) -> (x .and. y?=w387:bool)
    n303 = And(x=w333, y=w332) -> (x .and. y?=w330:bool)
    n304 = Subtract(x=w325, y=w331) -> (x-y=w329:dbl)
    n305 = And(x=w346, y=w345) -> (x .and. y?=w343:bool)
    n306 = Subtract(x=w336, y=w344) -> (x-y=w342:dbl)
    n307 = And(x=w359, y=w358) -> (x .and. y?=w356:bool)
    n308 = Subtract(x=w339, y=w357) -> (x-y=w355:dbl)
    n309 = case shown="True" w380 {
      tunnel: w381 -> [_ w533]
      tunnel: [0.0 w533] -> w370
      frame False {
      }
      frame True {
      }
    }
    n310 = case shown="True" w409 {
      tunnel: w408 -> [_ w537]
      tunnel: [0.0 w537] -> w402
      frame False {
      }
      frame True {
      }
    }
    n311 = case shown="False" w435 {
      tunnel: w434 -> [_ w545]
      tunnel: [0.0 w545] -> w432
      frame False {
      }
      frame True {
      }
    }
    n312 = case shown="False" w424 {
      tunnel: w425 -> [_ w541]
      tunnel: [0.0 w541] -> w415
      frame False {
      }
      frame True {
      }
    }
    n313 = case shown="True" w398 {
      tunnel: w399 -> [_ w525]
      tunnel: [0.0 w525] -> w362
      frame False {
      }
      frame True {
      }
    }
    n314 = case shown="True" w137 {
      tunnel: w136 -> [_ w457]
      tunnel: [0.0 w457] -> w115
      frame False {
      }
      frame True {
      }
    }
    n315 = case shown="True" w387 {
      tunnel: w386 -> [_ w529]
      tunnel: [0.0 w529] -> w363
      frame False {
      }
      frame True {
      }
    }
    n316 = case shown="True" w151 {
      tunnel: w152 -> [_ w461]
      tunnel: [0.0 w461] -> w116
      frame False {
      }
      frame True {
      }
    }
    n317 = case shown="True" w127 {
      tunnel: w128 -> [_ w453]
      tunnel: [0.0 w453] -> w114
      frame False {
      }
      frame True {
      }
    }
    n318 = case shown="True" w235 {
      tunnel: w234 -> [_ w485]
      tunnel: [0.0 w485] -> w198
      frame False {
      }
      frame True {
      }
    }
    n319 = case shown="True" w213 {
      tunnel: w212 -> [_ w477]
      tunnel: [0.0 w477] -> w196
      frame False {
      }
      frame True {
      }
    }
    n320 = case shown="True" w227 {
      tunnel: w228 -> [_ w481]
      tunnel: [0.0 w481] -> w197
      frame False {
      }
      frame True {
      }
    }
    n321 = case shown="True" w252 {
      tunnel: w253 -> [_ w489]
      tunnel: [0.0 w489] -> w199
      frame False {
      }
      frame True {
      }
    }
    n322 = case shown="True" w292 {
      tunnel: w291 -> [_ w501]
      tunnel: [0.0 w501] -> w283
      frame False {
      }
      frame True {
      }
    }
    n323 = case shown="True" w261 {
      tunnel: w260 -> [_ w493]
      tunnel: [0.0 w493] -> w200
      frame False {
      }
      frame True {
      }
    }
    n324 = case shown="True" w304 {
      tunnel: w303 -> [_ w505]
      tunnel: [0.0 w505] -> w284
      frame False {
      }
      frame True {
      }
    }
    n325 = case shown="True" w179 {
      tunnel: w178 -> [_ w469]
      tunnel: [0.0 w469] -> w158
      frame False {
      }
      frame True {
      }
    }
    n326 = case shown="True" w276 {
      tunnel: w277 -> [_ w497]
      tunnel: [0.0 w497] -> w201
      frame False {
      }
      frame True {
      }
    }
    n327 = case shown="True" w316 {
      tunnel: w315 -> [_ w509]
      tunnel: [0.0 w509] -> w285
      frame False {
      }
      frame True {
      }
    }
    n328 = case shown="True" w330 {
      tunnel: w329 -> [_ w513]
      tunnel: [0.0 w513] -> w322
      frame False {
      }
      frame True {
      }
    }
    n329 = case shown="True" w190 {
      tunnel: w189 -> [_ w473]
      tunnel: [0.0 w473] -> w159
      frame False {
      }
      frame True {
      }
    }
    n330 = case shown="True" w343 {
      tunnel: w342 -> [_ w517]
      tunnel: [0.0 w517] -> w323
      frame False {
      }
      frame True {
      }
    }
    n331 = case shown="True" w166 {
      tunnel: w165 -> [_ w465]
      tunnel: [0.0 w465] -> w157
      frame False {
      }
      frame True {
      }
    }
    n332 = case shown="False" w356 {
      tunnel: w355 -> [_ w521]
      tunnel: [0.0 w521] -> w349
      frame False {
      }
      frame True {
      }
    }
    n333 = Build Array(w349, w323, w322, w285, w284, w283) -> (w350:dbl[])
    "7 Hz" <- w350
    n334 = Build Array(w432, w415, w402, w370, w363, w362) -> (w430:dbl[])
    "6 Hz" <- w430
    n335 = Array Max & Min(array=w350) -> (max value=w113:dbl, max index (indices)=→"Max Index 7":i32)  [unwired: 2 out]
    "PSD max 7" <- w113
    n336 = Array Max & Min(array=w430) -> (max value=w110:dbl, max index (indices)=→"Max Index 6":i32)  [unwired: 2 out]
    "PSD max 6" <- w110
    n337 = Build Array(w201, w200, w199, w198, w197, w196) -> (w202:dbl[])
    "8 Hz" <- w202
    n338 = Build Array(w159, w158, w157, w116, w115, w114) -> (w160:dbl[])
    "9 Hz" <- w160
    n339 = Array Max & Min(array=w202) -> (max value=w112:dbl, max index (indices)=→"Max Index 8":i32)  [unwired: 2 out]
    "PSD max 8" <- w112
    n340 = Array Max & Min(array=w160) -> (max value=w111:dbl, max index (indices)=→"Max Index 9":i32)  [unwired: 2 out]
    "PSD max 9" <- w111
    n341 = Build Array(w110, w113, w112, w111) -> (w109:dbl[])
    n342 = Array Max & Min(array=w109) -> (max value=w107:dbl, max index (indices)=w108:i32)  [unwired: 2 out]
    "max value" <- w107
    "PSD MAX" <- w107
    n343 = Greater?(x=w107, y=0.0 ("x")) -> (0:w105:bool)
    n344 = case shown="False" w105 {
      tunnel: w108 -> [_ w451]
      tunnel: [555 w451] -> w94
      frame False {
      }
      frame True {
      }
    }
    "Index ที่มากที่สุด" <- w94
    n345 = Equal?(x=0, y=w94) -> (x = y?=→"6 HZ":bool)
    n346 = Equal?(x=1, y=w94) -> (x = y?=→"7 HZ":bool)
    n347 = Equal?(x=2, y=w94) -> (x = y?=→"9 HZ":bool)
    n348 = Equal?(x=3, y=w94) -> (x = y?=→"8 HZ":bool)
    n349 = Equal?(x=555, y=w94) -> (x = y?=→"555":bool)
  }
  n350 = while {
    stop <- FALSE stop-if-true
    n351 = event shown="[5] \"MENU 4\": Value Change" {
      selector: _ -> [_ _ _ _ _ _ _]
      dyn-events: _ -> [_ _ _ _ _ _ _]
      timeout: _ -> [_ _ _ _ _ _ _]
      event Timeout {
        n352 = event-data() -> ()  [unwired: 1 in, 3 out]
      }
      event "MENU": Value Change {
        n353 = event-data() -> ()  [unwired: 1 in, 6 out]
        n354 = local write "Tab Control"(enum32{"TAB 1", "TAB 2", "TAB 3", "TAB 4"}."TAB 2" ("Tab Control")) -> ()
      }
      event Value Change {
        n355 = event-data() -> ()  [unwired: 1 in, 6 out]
        n356 = local write "Tab Control"(enum32{"TAB 1", "TAB 2", "TAB 3", "TAB 4"}."TAB 1" ("Tab Control")) -> ()
      }
      event "MENU 2": Value Change {
        n357 = event-data() -> ()  [unwired: 1 in, 6 out]
        n358 = local write "Tab Control"(enum32{"TAB 1", "TAB 2", "TAB 3", "TAB 4"}."TAB 3" ("Tab Control")) -> ()
      }
      event "MENU 3": Value Change {
        n359 = event-data() -> ()  [unwired: 1 in, 6 out]
        n360 = local write "Tab Control"(enum32{"TAB 1", "TAB 2", "TAB 3", "TAB 4"}."TAB 4" ("Tab Control")) -> ()
      }
      event "MENU 4": Value Change {
        n361 = event-data() -> ()  [unwired: 1 in, 6 out]
        n362 = local write "Tab Control"(enum32{"TAB 1", "TAB 2", "TAB 3", "TAB 4"}."TAB 4" ("Tab Control")) -> ()
      }
      event "Back 4": Value Change {
        n363 = event-data() -> ()  [unwired: 1 in, 6 out]
        n364 = local write "Tab Control"(enum32{"TAB 1", "TAB 2", "TAB 3", "TAB 4"}."TAB 1" ("Tab Control")) -> ()
      }
    }
  }
  n365 = while {
    shift-right: [w564] -> _
    shift-left: "" -> [w566]
    stop <- FALSE stop-if-true
    n366 = event shown="[0] \"Text1\": Value Change" {
      selector: _ -> [_ _ _]
      dyn-events: _ -> [_ _ _]
      timeout: _ -> [_ _ _]
      tunnel: w566 -> [_ _ _]
      tunnel: ["ช่วยด้วย ฉันต้องการความช่วยเหลือ !!!" "ฉันต้องการรับประทานอาหาร" "ฉันมีโรคประจำตัว และรู้สึกอาการกำเริบ !!!"] -> w564
      event "Text1": Value Change {
        n367 = event-data() -> ()  [unwired: 1 in, 6 out]
      }
      event "Text2": Value Change {
        n368 = event-data() -> ()  [unwired: 1 in, 6 out]
      }
      event "Text3": Value Change {
        n369 = event-data() -> ()  [unwired: 1 in, 6 out]
      }
    }
    "String" <- w564
  }
  n370 = call-poly "VISA Configure Serial Port"("VISA resource name"="VISA resource name", "baud rate (9600)"=u32 9600) -> ("VISA resource name out"=w7:refnum<visa-resource-name>, "error out"=w5:errorcluster)  [unwired: 12 in]
  n371 = while {
    shift-right: [w578] -> w6
    shift-left: w7 -> [w579]
    shift-right: [w576] -> w4
    shift-left: w5 -> [w577]
    stop <- FALSE stop-if-true
    n372 = Select(t="a", s="LED", f="b") -> (s? t:f=w573:string)
    n373 = VISA Write(VISA resource name=w579, write buffer=w573, error in (no error)=w577) -> (VISA resource name out=w578:refnum<visa-resource-name>, error out=w576:errorcluster)  [unwired: 1 out]
    n374 = Wait (ms)(milliseconds to wait=u32 5) -> ()  [unwired: 1 out]
  }
  n375 = VISA Close(VISA resource name=w6, error in (no error)=w4) -> ()  [unwired: 1 out]
